vi "Build Connection Array from string.vi"(11 "Connection String":string="water-to-light map:\n88 18 7\n18 25 70") -> (3 "Range Cluster":T1[](array[typedef]))   [LabVIEW 2023]
uses:
  Cluster_Sorce Destination Connection.ctl
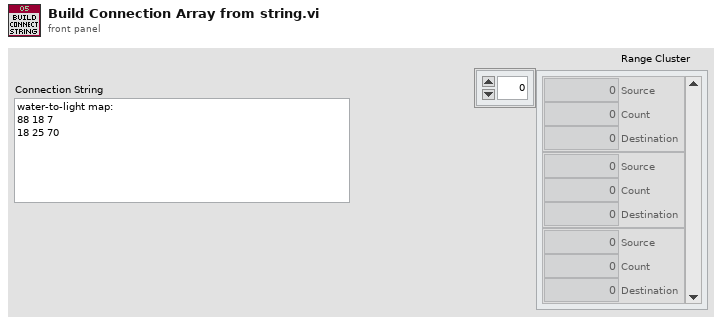
[diagram p1: front panel]
types:
  T1 = typedef "Cluster_Sorce Destination Connection.ctl" = cluster{"Source":i64, "Count":i64, "Destination":i64}
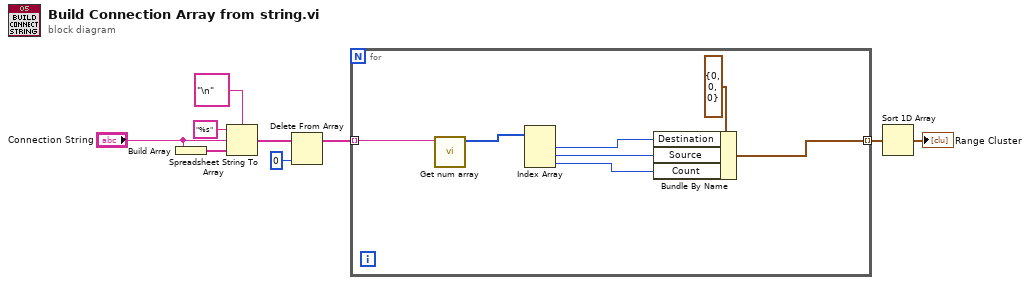
[diagram p0: block diagram]
diagram:
  n1 = Build Array("Connection String") -> (w9:string[])
  n2 = Spreadsheet String To Array(delimiter (Tab)="\n", format string="%s", spreadsheet string="Connection String", array type (2D Dbl)=w9) -> (array=w6:string[])
  n3 = Delete From Array(array=w6, index=0) -> (array with subset deleted=w3:string[])  [unwired: 1 in, 1 out]
  n4 = for {
    tunnel: w3 -> [w16] mode=indexing
    tunnel: [w13] -> w2 mode=indexing
    n5 = call "Get num array.vi"("number String"=w16) -> ("number Array"=w15:i64[])  [unwired: 10 in]
    n6 = Index Array(array=w15) -> (element #1=w12:i64, element #2=w11:i64, element #3=w10:i64)  [unwired: 3 in]
    n7 = Bundle By Name(cluster=T1 {"Source"=0, "Count"=0, "Destination"=0} ("Source Destination Connect"), "Destination"=w12, "Source"=w11, "Count"=w10) -> (w13:T1)
  }
  n8 = Sort 1D Array(array=w2) -> (sorted array=→"Range Cluster":T1[])
